vi "Oscilloscpe.vi"() -> ()   [LabVIEW 2011]
uses:
  <instrlib>/Tektronix DPO MSO 2000 4000 Series/Public/Data/Read (Multiple Waveforms).vi
  <vilib>/express/express analysis/Spectral/Block/exnSpectralBlock spectral measurements RMS poly.vi
  <vilib>/express/express analysis/Spectral/Block/exnSpectralBlock spectral measurements RMS array WFM.vi
  <vilib>/express/express analysis/Spectral/XNode/ExpressSpectralMeasurementsBlockNode.xnode
  <vilib>/Waveform/WDTFileIO.llb/Export Waveforms To Spreadsheet File (1D).vi
  <vilib>/Analysis/baseanly.llb/IIR Cascade Filter (DBL).vi
  <instrlib>/Tektronix DPO MSO 2000 4000 Series/Tektronix DPO MSO 2000 4000 Series.lvlib
  <vilib>/Analysis/NI_AALBase.lvlib
panel:
  out "Waveform Graph 2":dbl[](graph)
  out "path":path
  in  "Name of File":string
  in  "stop":bool
  out "Channel 1":waveform(dbl)[](graph)
  out "Channel1 FFT":cluster{"f0":dbl, "df":dbl, "magnitude":dbl[]}[](graph)
  out "Channel 2":waveform(dbl)[](graph)
  out "Channel 2 FFT":cluster{"f0":dbl, "df":dbl, "magnitude":dbl[]}[](graph)
  in  "VISA resource name":refnum<visa-resource-name>
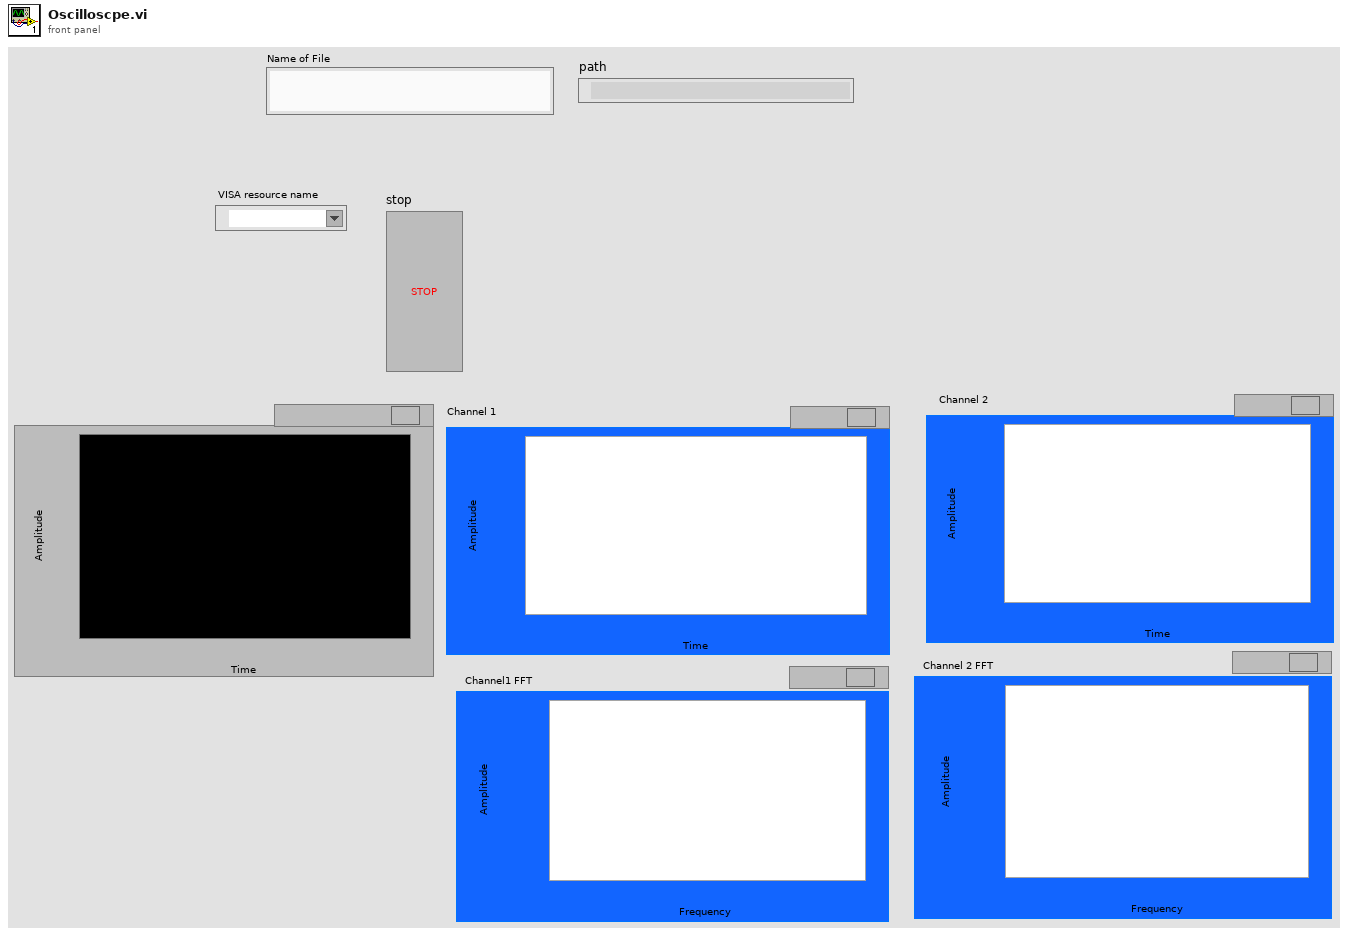
[diagram p1: front panel]
types:
  T1 = enum16{"open", "replace", "create", "open or create", "replace or create", "replace or create with confirmation"}
  T2 = cluster{"averaging mode":u16, "weighting mode":u16, "number of averages":u32}
  T3 = cluster{"dB On (F)":bool, "unwrap phase (F)":bool, "convert to degree (F)":bool}
  T4 = cluster{"filter structure":enum32{"IIR 2nd Order", "IIR 4th Order"}, "Reverse Coefficients":dbl[], "Forward Coefficients":dbl[]}
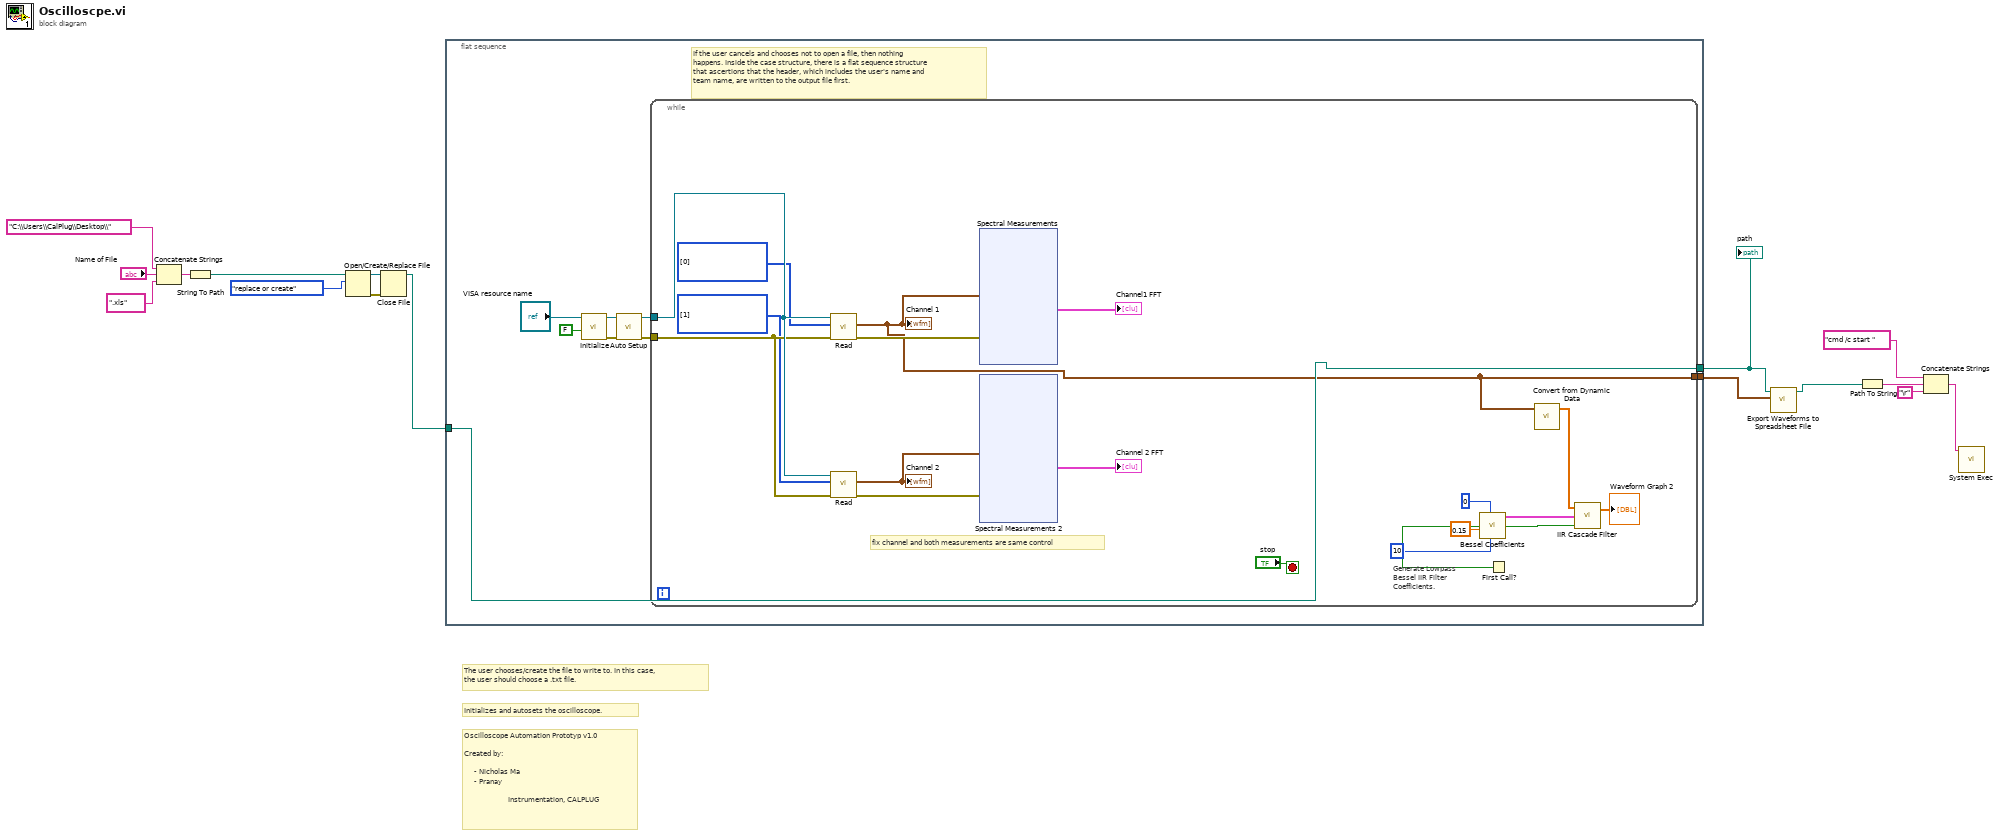
[diagram p0: block diagram]
diagram:
  # "Initializes and autosets the oscilloscope."
  # "The user chooses/create the file to write to. In this case, \nthe user should choose a .txt file."
  # "Oscilloscope Automation Prototyp v1.0\n\nCreated by:\n     \n     - Nicholas Ma\n     - Pranay\n\n                      Instrumentation, CALPLUG"
  n1 = Concatenate Strings("C:\\Users\\CalPlug\\Desktop\\" ("string"), "Name of File", ".xls" ("string")) -> (w16:string)
  n2 = String To Path(string=w16) -> (path=w15:path)
  n3 = Open/Create/Replace File(file path (use dialog)=w15, operation (0:open)=T1."replace or create") -> (refnum out=w10:refnum<file>, error out=w9:errorcluster)  [unwired: 4 in, 1 out]
  n4 = Close File(refnum=w10, error in=w9) -> (path=w8:path)  [unwired: 1 out]
  n5 = flat-sequence {
    tunnel: w8 -> [w18]
    tunnel: [w18] -> w3
    tunnel: [w17] -> w1
    frame #0 {
      # "If the user cancels and chooses not to open a file, then nothing\nhappens. Inside the case structure, there is a flat sequence structure\nthat ascertions that the header, which includes the user's name and\nteam name, are written to the output file first."
      n6 = call <instrlib>:"Initialize.vi"("Reset (True)"=FALSE, "VISA resource name"="VISA resource name") -> ("error out"=w24:errorcluster, "VISA resource name out"=w23:refnum<visa-resource-name>)  [unwired: 8 in]
      n7 = call <instrlib>:"Auto Setup.vi"("error in (no error)"=w24, "VISA resource name"=w23) -> ("error out"=w19:errorcluster, "VISA resource name out"=w20:refnum<visa-resource-name>)  [unwired: 8 in]
      n8 = while {
        tunnel: w20 -> [w41]
        tunnel: w19 -> [w40]
        tunnel: [w25] -> w17
        stop <- "stop" stop-if-true
        w37 = u16[] [0] items=["Channel 1", "Channel 2", "Channel 3", "Channel 4", "Math", "Reference 1", "Reference 2", "Reference 3", "Reference 4"] ("Channels")
        w34 = u16[] [1] items=["Channel 1", "Channel 2", "Channel 3", "Channel 4", "Math", "Reference 1", "Reference 2", "Reference 3", "Reference 4"] ("Channels")
        # "Generate Lowpass\nBessel IIR Filter \nCoefficients."
        # "fix channel and both measurements are same control"
        n9 = call-poly <instrlib>:"Read.vi"("error in (no error)"=w40, "Channels"=w37, "VISA resource name"=w41) -> ("error out"=w39:errorcluster, "Waveform Data"=w25:waveform(dbl)[])  [unwired: 6 in, 1 out]
        "Channel 1" <- w25
        n10 = call-poly <instrlib>:"Read.vi"("error in (no error)"=w40, "Channels"=w34, "VISA resource name"=w41) -> ("error out"=w36:errorcluster, "Waveform Data"=w33:waveform(dbl)[])  [unwired: 6 in, 1 out]
        "Channel 2" <- w33
        n11 = xnode "Spectral Measurements"("Signals"=w25, "error in (no error)"=w39) -> ("FFT - (RMS)"=→"Channel1 FFT":cluster{"f0":dbl, "df":dbl, "magnitude":dbl[]}[])  [unwired: 2 out]
        n12 = xnode "Spectral Measurements 2"("Signals"=w33, "error in (no error)"=w36) -> ("FFT - (RMS)"=→"Channel 2 FFT":cluster{"f0":dbl, "df":dbl, "magnitude":dbl[]}[])  [unwired: 2 out]
        n13 = call <vilib>:"Bessel Coefficients.vi"("order"=10, "filter type"=0, "low cutoff freq: fl"=0.15) -> ("IIR Filter Cluster"=w27:T4)  [unwired: 7 in, 1 out]
        n14 = First Call?() -> (First Call?: T/F=w30:bool)
        n15 = call "Convert from Dynamic Data"("Dynamic Data Type"=w25) -> ("Array"=w31:dbl[])  [unwired: 3 in]
        n16 = call-poly <vilib>:"IIR Cascade Filter.vi"("init/cont (init:F)"=w30, "IIR Filter Cluster"=w27, "X"=w31) -> ("Filtered X"=→"Waveform Graph 2":dbl[])  [unwired: 1 out]
      }
    }
  }
  n17 = call-poly <vilib>:"Export Waveforms to Spreadsheet File.vi"("waveforms"=w1, "file path (dialog if empty)"=w3) -> ("new file path (Not A Path if cancelled)"=w2:path)  [unwired: 8 in, 1 out]
  n18 = Path To String(path=w2) -> (string=w5:string)
  n19 = Concatenate Strings("cmd /c start " ("string"), w5, "\r") -> (w6:string)
  n20 = call <vilib>:"System Exec.vi"("command line"=w6) -> ()  [unwired: 7 in, 4 out]
  "path" <- w3
